vi "State Data.vi"(11 "Display State In":cluster{"Month":i32, "Day":i32, "Year":i32}) -> (3 "Data Out":string)   [LabVIEW 2019, in "Custom Calendar.xctl"]
uses:
  Custom Calendar.xctl
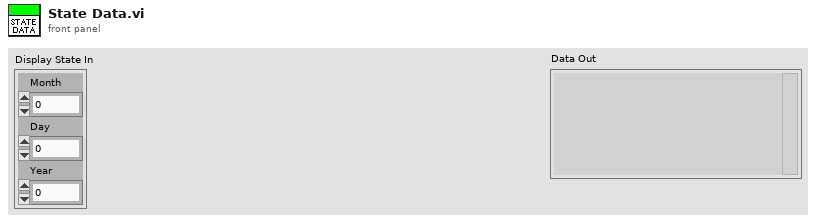
[diagram p1: front panel]
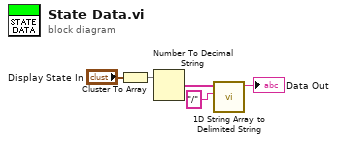
[diagram p0: block diagram]
diagram:
  n1 = Cluster To Array(cluster="Display State In") -> (array=w4:i32[])
  n2 = Number To Decimal String(number=w4) -> (decimal integer string=w3:string[])  [unwired: 1 in]
  n3 = call <vilib>:"1D String Array to Delimited String.vi"("delimiter"="/", "string array"=w3) -> ("delimited string"=→"Data Out":string)  [unwired: 9 in]
